vi "Release-parameter-refs.vi"(8 "error in (no error)":errorcluster, 11 "Data ref. in":refnum<data-value>) -> (0 "error out":errorcluster, 3 "Data ref.":refnum<data-value>)   [LabVIEW 2013, in "CameraVision.lvlib" / "CV-Main.lvclass"]
uses:
  CV-Main.lvclass
  CV-Main.lvclass/CV-Main.ctl
  Acquisition/CV-Acquisition.lvclass
  Analysis/CV-Analysis.lvclass
  Configuration/CV-Configuration.lvclass
  Correction/CV-Correction.lvclass
  Mapping/CV-Mapping.lvclass
  Storage/CV-Storage.lvclass
  Temperature/CV-Temperature.lvclass
  Filter/CV-Filter.lvclass
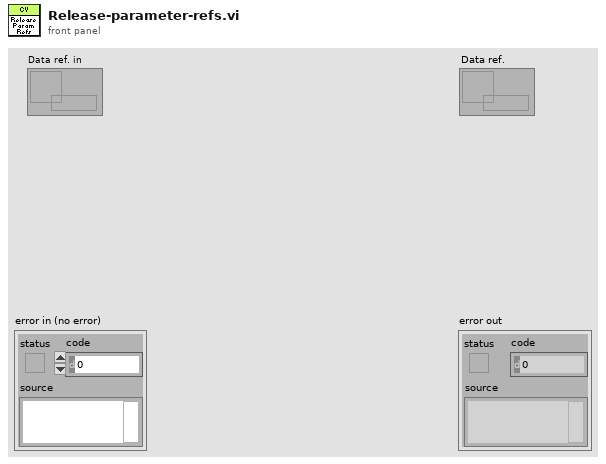
[diagram p1: front panel]
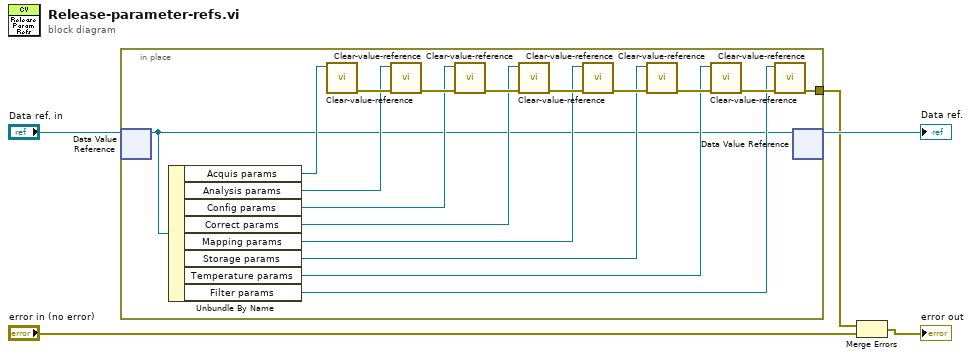
[diagram p0: block diagram]
diagram:
  n1 = in-place {
    in-place-border: [w7] -> w1
    n2 = in-place-dvr #1("Data ref. in") -> (w6:refnum<class "CV-Main.lvclass">)  [unwired: 1 out]
    n3 = Unbundle By Name(w6) -> ("Acquis params"=w13:refnum<data-value>, "Analysis params"=w15:refnum<data-value>, "Config params"=w14:refnum<data-value>, "Correct params"=w12:refnum<data-value>, "Mapping params"=w11:refnum<data-value>, "Storage params"=w10:refnum<data-value>, "Temperature params"=w9:refnum<data-value>, "Filter params"=w8:refnum<data-value>)
    n4 = call "Clear-value-reference.vi"("Acquis. params. ref."=w13) -> ("error out"=w22:errorcluster)  [unwired: 9 in, 1 out]
    n5 = call "Clear-value-reference.vi"("error in (no error)"=w22, "Analysis params. ref."=w15) -> ("error out"=w21:errorcluster)  [unwired: 8 in, 1 out]
    n6 = call "Clear-value-reference.vi"("error in (no error)"=w21, "Config. params. ref."=w14) -> ("error out"=w20:errorcluster)  [unwired: 8 in, 1 out]
    n7 = call "Clear-value-reference.vi"("error in (no error)"=w20, "Correct. params. ref."=w12) -> ("error out"=w19:errorcluster)  [unwired: 8 in, 1 out]
    n8 = call "Clear-value-reference.vi"("error in (no error)"=w19, "Mapping params. ref."=w11) -> ("error out"=w18:errorcluster)  [unwired: 8 in, 1 out]
    n9 = call "Clear-value-reference.vi"("error in (no error)"=w18, "Storage params. ref."=w10) -> ("error out"=w17:errorcluster)  [unwired: 8 in, 1 out]
    n10 = call "Clear-value-reference.vi"("error in (no error)"=w17, "Temp. params. ref."=w9) -> ("error out"=w16:errorcluster)  [unwired: 8 in, 1 out]
    n11 = call "Clear-value-reference.vi"("error in (no error)"=w16, "Filter params. ref."=w8) -> ("error out"=w7:errorcluster)  [unwired: 8 in, 1 out]
    n12 = in-place-dvr #1(w6) -> (→"Data ref.":refnum<data-value>)  [unwired: 1 out]
  }
  n13 = Merge Errors(w1, "error in (no error)") -> (→"error out":errorcluster)
